vi "Find Average Center_10152025.vi"(5 "Position":i32, 7 "Tray Number":i32, 8 "Assembly Type":string, 9 "XYZTheta":dbl[](array[numeric]), 11 "Gantry In":refnum<k24>) -> (1 "XYZTheta":dbl[](array[numeric]) format="%.6g", 3 "Gantry Out":refnum<k24>)   [LabVIEW 2021, in "Component Tray.lvclass"]
uses:
  Component Tray.lvclass
  Find Component.ctl
  Controller/Camera/Machine Vision.ctl
  C:/Program Files (x86)/Aerotech/A3200/LabVIEW/2010/Bin/Aerotech.A3200.dll
  Program Files (x86)/Aerotech/A3200/LabVIEW/2010/Bin/Aerotech.A3200.dll
  Controller/Camera/Image processing.ctl
  Controller/Camera/Camera settings.ctl
  <vilib>/vision/Pattern Matching.llb/IMAQ GM Match Report.ctl
  Controller/Camera/Edmund Optics/Edmund Optics.lvclass
  C:/Users/HEP/Documents/GitHub/Gantry/UCSB-Gantry-HEP-main/Classes/Controller/Camera/Camera.lvclass
  <vilib>/picture/picture.llb/imagedata.ctl
  Controller/Camera/Camera.lvclass
  Controller/Motion/A3200/A3200.lvclass
  Controller/Motion/Motion.lvclass
panel:
  out "pattern matching":T1 {"Correlation Score" format="%.2f"; "Target Template Curve Score" format="%.2f"; "Template Target Curve Score" format="%.2f"; "Bounding Box"."y" format="%.2f"; "Bounding Box"."x" format="%.2f"; "Position"."y" format="%.2f"; "Position"."x" format="%.2f"; "Score" format="%.2f"; "Scale" format="%.2f"; "Angle" format="%.2f"; "Occlusion %" format="%.2f"}
  out "Maximal Value":sgl
  out "Standard Variation":sgl
  out "Match found?":bool
  out "Radius (Real-World)":dbl
  in  "Enter Manual Mode":bool
  out "Manual Mode On":bool
  in  "Auto Submit":bool
  out "Instructions":string="Use the joystick to match the pattern recognition until a red circle appears.\nUse Z controls to focus if needed."
  out "Tray and Position":string
  out "Sensor ID":picture[](array[picture])
  out "Sensor ID":string
  in  "Machine Vision":T2
  out "predicted fiducials":dbl[][](array[numeric])
  out "Current Z High Speed":dbl
  out "Current XY High Speed":dbl
  out "current Z low speed":dbl
  out "current XY speed":dbl
  in  "Z high":dbl=12.5
  in  "XY high":dbl=50.0
  in  "Z low":dbl=0.05
  in  "XY low":dbl=0.1
  in  "Predict fiducials":bool
  out "Low Speed":bool
  out "X":bool
  out "Y":bool
  out "Z":bool
  out "High Speed":bool
  in  "Go to CH191/FD5":bool
  in  "Go to CH197/FD4":bool
  out "Program Stopped":bool
  out "XY Graph":cluster{"X":dbl, "Y":dbl}[](graph)
  out "Sensor ID Location":dbl[](array[numeric])
  in  "Go to Sensor ID":bool
  out "CH1 XYZ":dbl[](array[numeric])
  out "CH1 correct?":bool
  in  "Go to CH1":bool
  in  "Focus step size":dbl format="%#_13g"
  in  "number of focus steps":i32
  out "Average Strength":dbl
  in  "Focus":bool
  out "All fiducials recorded":bool
  in  "Override presets":bool
  in  "Camera settings":T3={"Gamma"=1.6, "Gain"=0, "Sharpness"=0, "Contrast"=0.0, "Exposure"=0.0078125} {"Exposure" min=0.000244140625 max=0.5 scale=0.0002..0.5; "Contrast" min=0.0 max=1.0 scale=0.001..1.0; "Sharpness" min=0 max=2 step=1 scale=0.0..2.0; "Gain" min=0 max=100 step=1 scale=0.1..100.0; "Gamma" min=0.01 max=10.0 scale=0.01..10.0}
  in  "Image processing":T4={"Brightness"=128.0, "Contrast"=45.0, "Gamma"=1.0471123} {"Brightness" scale=0.0..400.0; "Contrast" scale=0.0..90.0; "Gamma" scale=0.005..5.0}
  out "Gantry":dbl[](array[numeric]) format="%.6g"
  out "Sum":dbl[](array[numeric]) format="%.6g"
  out "CH197/FD4 XYZ":dbl[](array[numeric]) format="%.6g"
  out "CH8/FD2 XYZ":dbl[](array[numeric]) format="%.6g"
  out "CH191/FD5 XYZ":dbl[](array[numeric]) format="%.6g"
  out "CH1/FD1 XYZ":dbl[](array[numeric]) format="%.6g"
  in  "Record CH8/FD2":bool
  in  "Record CH197/FD4":bool
  in  "Record CH191/FD5":bool
  in  "Record CH1/FD1":bool
  in  "Go to CH8/FD2":bool
  in  "Go to CH1/FD1":bool
  in  "Joystick":bool
  out "Camera":dbl[](array[numeric]) format="%.6g"
  in  "Go to Center":bool
  in  "Component":T5
  in  "Stop Program":bool
  out "Image":T6(plugin-control)
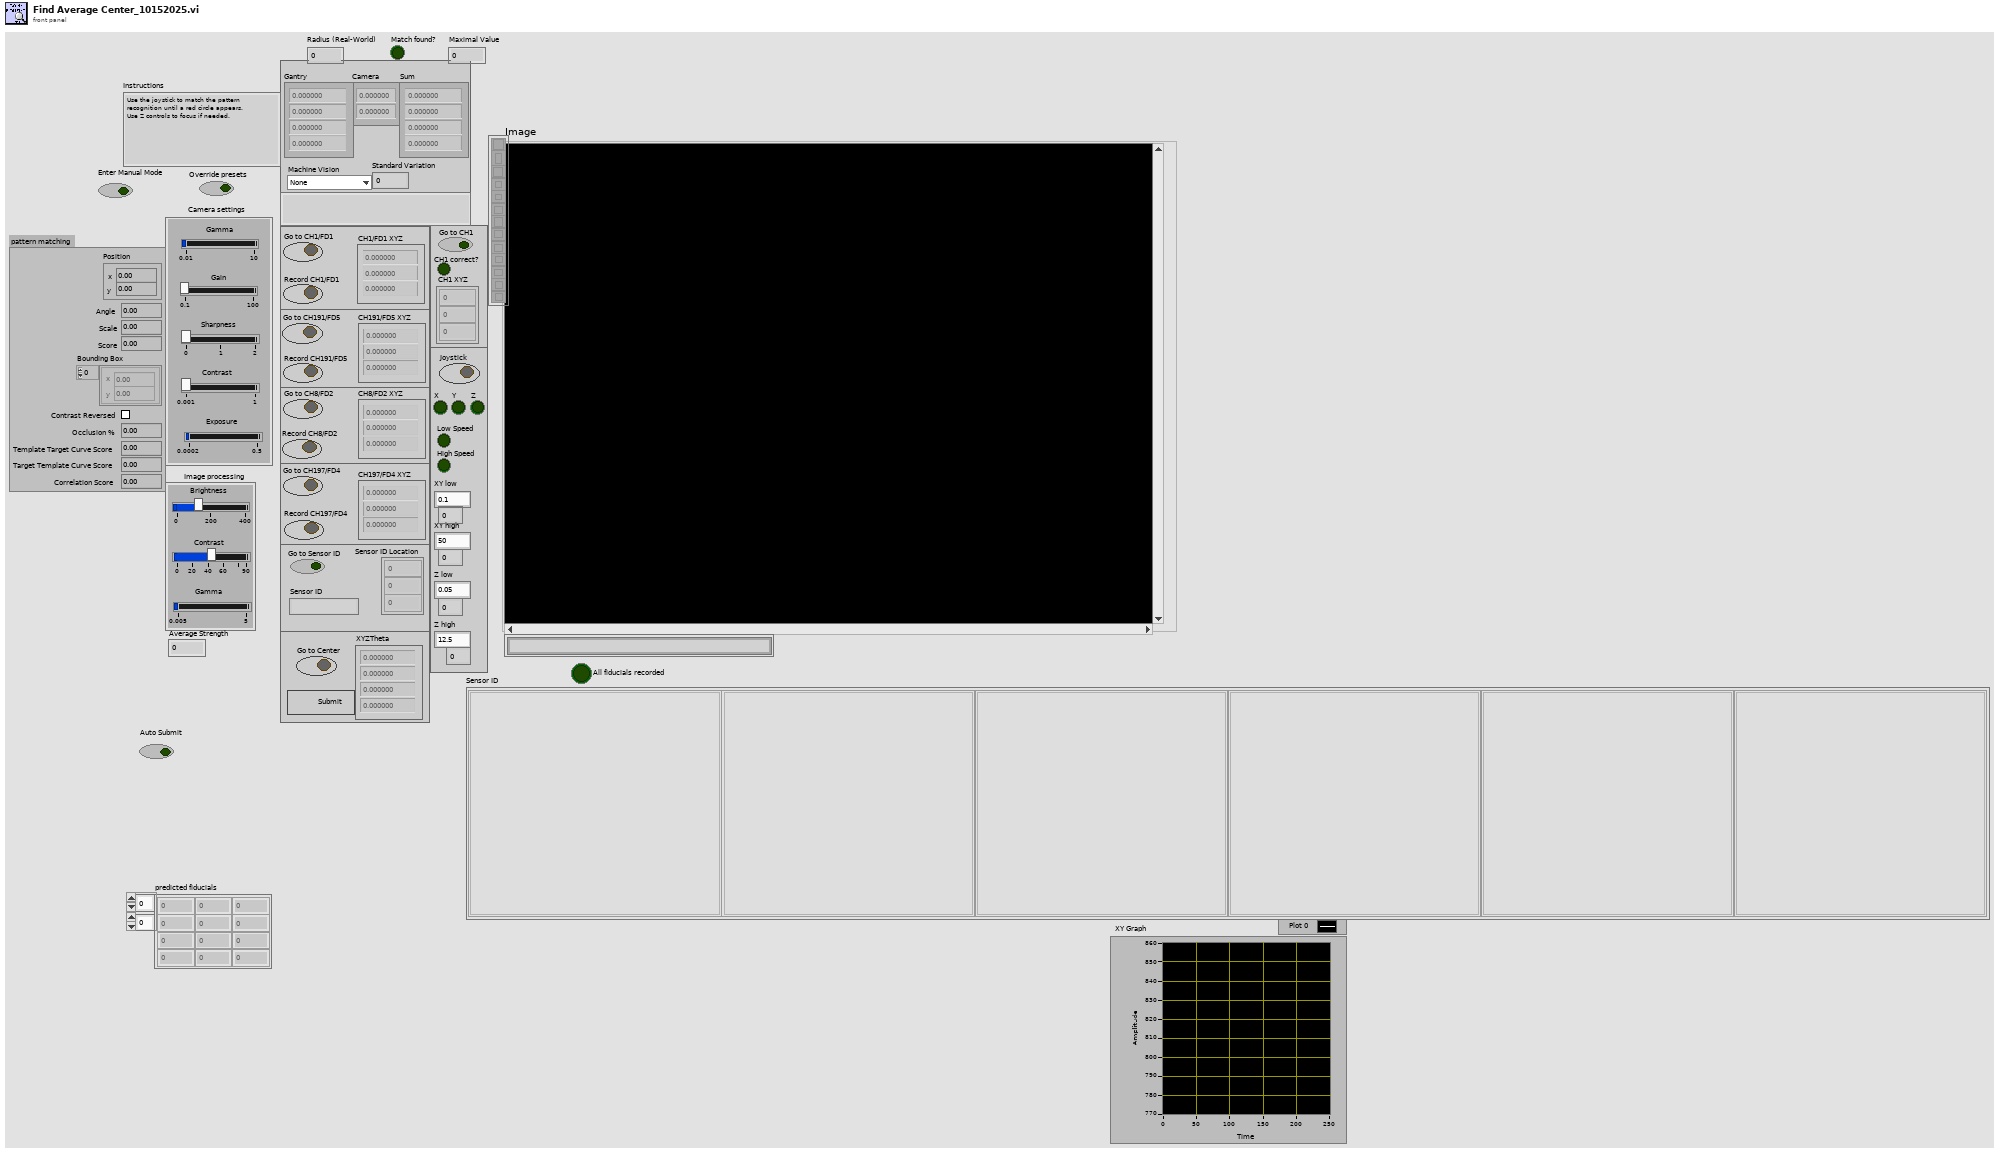
[diagram p1: front panel]
types:
  T1 = typedef "IMAQ GM Match Report.ctl" = cluster{"Position":cluster{"x":sgl, "y":sgl}, "Angle":sgl, "Scale":sgl, "Score":sgl, "Bounding Box":cluster{"x":sgl, "y":sgl}[], "Contrast Reversed":bool, "Occlusion %":sgl, "Template Target Curve Score":sgl, "Target Template Curve Score":sgl, "Correlation Score":sgl}
  T2 = typedef "Camera.lvclass/Machine Vision.ctl" = enum16{"None", "Tray Fiducials", "Sensor Fiducial", "V3 Sensor Circle", "Partial Hexaboard", "Hexaboard Circle", "sensor CH1 check", "sensor edge pos1", "sensor edge pos2", "HB edge pos1", "HB edge pos2", "HB Fiducial", "HB CH1 check "}
  T3 = typedef "Camera.lvclass/Camera settings.ctl" = cluster{"Gamma":dbl, "Gain":i64, "Sharpness":i64, "Contrast":dbl, "Exposure":dbl}
  T4 = typedef "Camera.lvclass/Image processing.ctl" = cluster{"Brightness":sgl, "Contrast":sgl, "Gamma":sgl}
  T5 = typedef "Component Tray.lvclass/Find Component.ctl" = cluster{"New Fiducials":dbl[], "Past Fiducials":dbl[][], "XYZTheta":dbl[], "Fiducials Path":path, "Position":i32, "CH1 Location":dbl[], "Sensor ID Location":dbl[], "raw rotation":dbl, "initial rotation":dbl[], "CH2":dbl[], "initial edge XYZ":dbl[], "max std variation":dbl, "max strength":dbl, "Pattern Matching":T2, "Fiducial Circle":T2, "Initial Edge":T2, "Pos multiplier":dbl, "time to wait":u32, "fiducial to edge":dbl, "Protomodule?":bool, "Assembly Type":string}
  T6 = typedef "IMAQ Image.ctl" = refnum<image>
  T7 = enum8{"Enabled", "Disabled", "Disabled and Grayed Out"}
  T8 = cluster{"left":i16, "top":i16, "right":i16, "bottom":i16}
  T9 = typedef "imagedata.ctl" = cluster{"image type":i32, "image depth":i32, "image":u8[], "mask":u8[], "colors":u32[], "Rectangle":cluster{"left":i16, "top":i16, "right":i16, "bottom":i16}}
  T10 = typedef "File Paths.ctl" = cluster{"Glue Pattern Folder":path, "Carrier Tray Folder":path, "Pick Up Tool Fixture Folder":path, "Components Folder":path, "Bellows Tool Offset.txt":path, "Pick Up Tool Offset.txt":path, "Dispense Tip Offset.txt":path, "Log Files":path, "Gantry Assembly Map.txt":path, "Syringe and offset map.txt":path, "Controllers Folder":path, "Local dbase config":path}
  T11 = cluster{"left":dbl, "top":dbl, "right":dbl, "bottom":dbl}
  T12 = cluster{"Average Strength":dbl, "Radius (Real-World)":dbl, "Match found?":bool, "initial angle":sgl, "Global Report":cluster{"Mean Value":sgl, "Standard Variation":sgl, "Minimal Value":sgl, "Maximal Value":sgl, "Area (calibrated)":sgl, "Area (pixels)":u32, "%":sgl, "Calibration Valid":bool}}
  T13 = cluster{"Mean Value":sgl, "Standard Variation":sgl, "Minimal Value":sgl, "Maximal Value":sgl, "Area (calibrated)":sgl, "Area (pixels)":u32, "%":sgl, "Calibration Valid":bool}
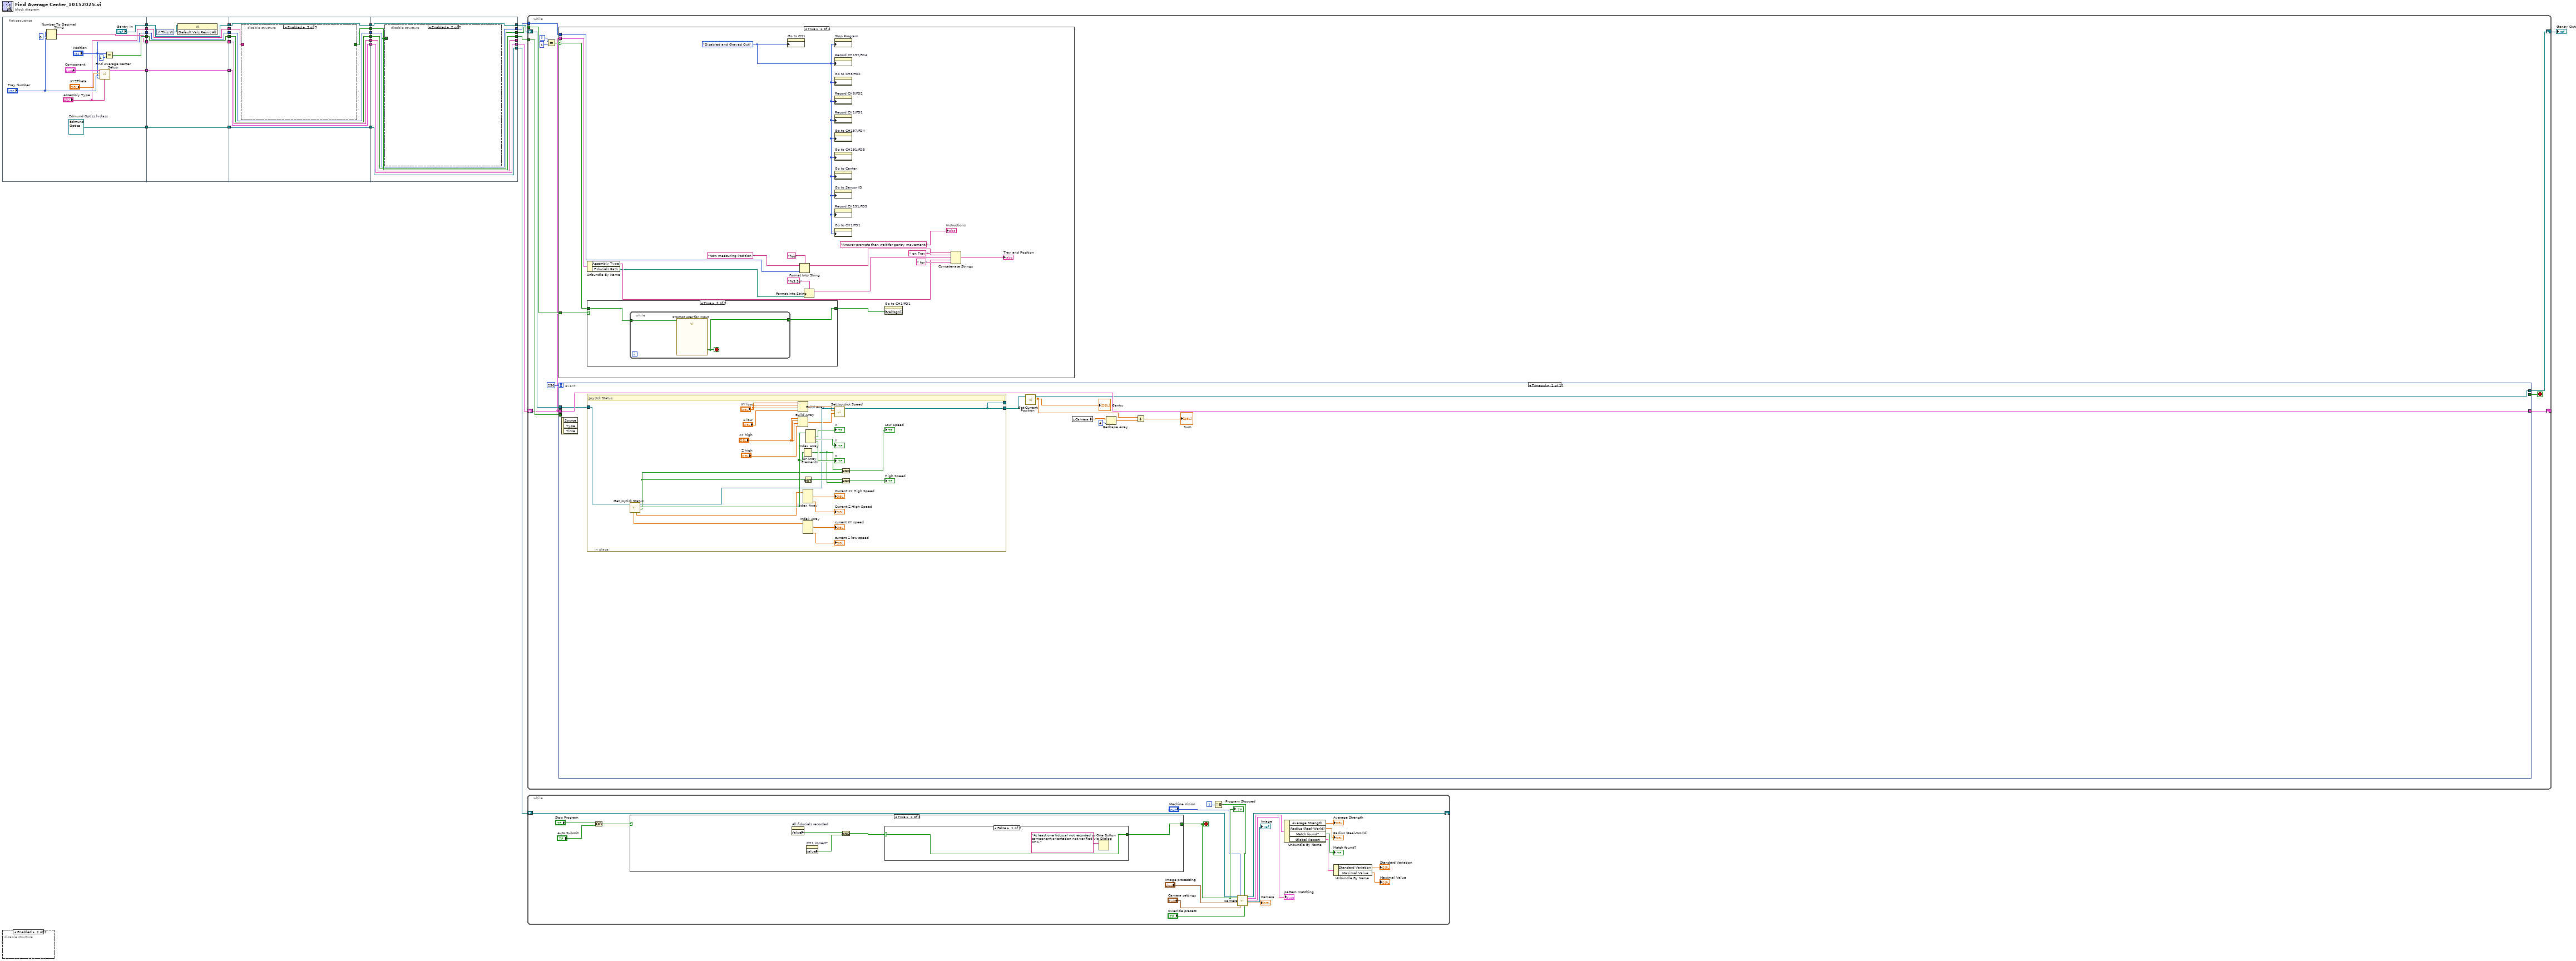
[diagram p0: block diagram]
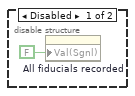
[diagram p2: hidden frame]
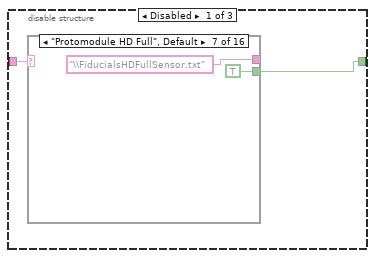
[diagram p3: hidden frame]
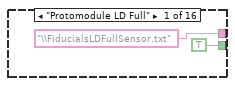
[diagram p4: hidden frame]
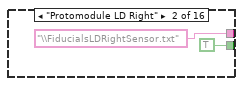
[diagram p5: hidden frame]
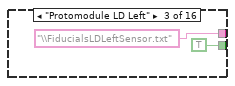
[diagram p6: hidden frame]
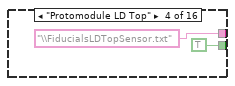
[diagram p7: hidden frame]
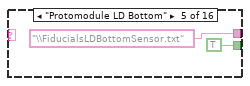
[diagram p8: hidden frame]
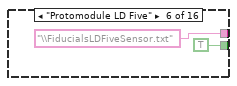
[diagram p9: hidden frame]
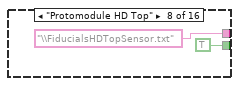
[diagram p10: hidden frame]
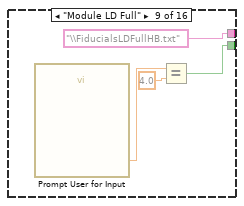
[diagram p11: hidden frame]
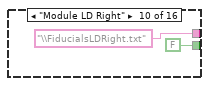
[diagram p12: hidden frame]
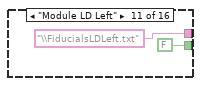
[diagram p13: hidden frame]
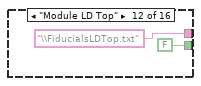
[diagram p14: hidden frame]
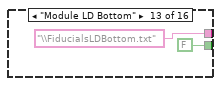
[diagram p15: hidden frame]
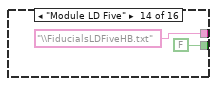
[diagram p16: hidden frame]
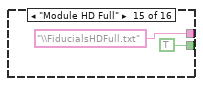
[diagram p17: hidden frame]
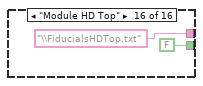
[diagram p18: hidden frame]
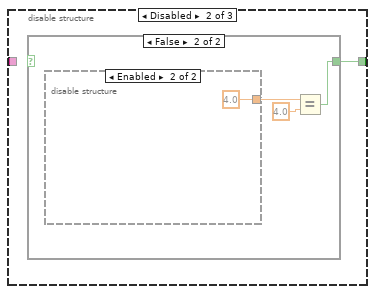
[diagram p19: hidden frame]
diagram:
  n1 = flat-sequence {
    tunnel: [w33] -> w23
    tunnel: [w37] -> w19
    tunnel: ["Gantry In"] -> w15
    tunnel: [w36] -> w12
    tunnel: ["Position"] -> w8
    tunnel: [w35] -> w5
    tunnel: ["Assembly Type"] -> w2
    tunnel: [w47] -> w24
    tunnel: w23 -> [w47]
    tunnel: [w46] -> w20
    tunnel: w19 -> [w46]
    tunnel: [w45] -> w16
    tunnel: w15 -> [w45]
    tunnel: [w44] -> w13
    tunnel: w12 -> [w44]
    tunnel: [w43] -> w9
    tunnel: w8 -> [w43]
    tunnel: w5 -> [w42]
    tunnel: [w42] -> w3
    tunnel: w2 -> [w41]
    tunnel: [w41] -> w1
    tunnel: [w56] -> w27
    tunnel: [w55] -> w25
    tunnel: w24 -> [w55]
    tunnel: [w54] -> w21
    tunnel: w20 -> [w54]
    tunnel: [w53] -> w17
    tunnel: w16 -> [w53]
    tunnel: w13 -> [w52]
    tunnel: [w52] -> w11
    tunnel: w9 -> [w51]
    tunnel: [w51] -> w7
    tunnel: [w50] -> w4
    tunnel: w3 -> [w50]
    tunnel: w1 -> [w49]
    tunnel: w27 -> [w106]
    tunnel: [w106] -> w26
    tunnel: [w105] -> w22
    tunnel: w25 -> [w105]
    tunnel: w21 -> [w104]
    tunnel: [w104] -> w18
    tunnel: [w103] -> w14
    tunnel: w17 -> [w103]
    tunnel: w11 -> [w102]
    tunnel: [w102] -> w10
    tunnel: [w101] -> w6
    tunnel: w7 -> [w101]
    tunnel: w4 -> [w100]
    tunnel: [w100] -> _
    frame #0 {
      w37 = refnum<class "Edmund Optics.lvclass"> refnum  # Edmund Optics.lvclass
      n2 = Number To Decimal String(number="Tray Number", width (-)=i16 0) -> (decimal integer string=w35:string)
      n3 = call "Find Average Center Setup.vi"("Assembly Type"="Assembly Type", "Position"="Position", "Tray Number"="Tray Number", "XYZTheta"="XYZTheta", "Component"="Component") -> ("output cluster"=w33:T5)  [unwired: 6 in]
      n4 = Equal?(x="Position", y=1) -> (x = y?=w36:bool)
    }
    frame #1 {
      n5 = control-ref of="This VI"() -> (w48:refnum<vi>)
      n6 = invoke class="VI" method="Default Vals.Reinit All"(reference=w48) -> ()  [unwired: 2 in, 3 out]
    }
    frame #2 {
      n7 = disable-structure shown="Enabled" {
        disable-tunnel: [w58 w93 _] -> w56
        disable-tunnel: w49 -> [w57 _ _]
        frame Disabled {
          n8 = case shown="\"Protomodule HD Full\", Default" w57 {
            tunnel: ["\\FiducialsLDFullSensor.txt" ("string") "\\FiducialsLDRightSensor.txt" ("string") "\\FiducialsLDLeftSensor.txt" ("string") "\\FiducialsLDTopSensor.txt" ("string") "\\FiducialsLDBottomSensor.txt" ("string") "\\FiducialsLDFiveSensor.txt" ("string") "\\FiducialsHDFullSensor.txt" ("string") "\\FiducialsHDTopSensor.txt" ("string") "\\FiducialsLDFullHB.txt" ("string") "\\FiducialsLDRight.txt" ("string") "\\FiducialsLDLeft.txt" ("string") "\\FiducialsLDTop.txt" ("string") "\\FiducialsLDBottom.txt" ("string") "\\FiducialsLDFiveHB.txt" ("string") "\\FiducialsHDFull.txt" ("string") "\\FiducialsHDTop.txt" ("string")] -> _
            tunnel: [TRUE TRUE TRUE TRUE TRUE TRUE TRUE TRUE w75 FALSE FALSE FALSE FALSE FALSE TRUE FALSE] -> w58
            frame "Protomodule LD Full" {
            }
            frame "Protomodule LD Right" {
            }
            frame "Protomodule LD Left" {
            }
            frame "Protomodule LD Top" {
            }
            frame "Protomodule LD Bottom" {
            }
            frame "Protomodule LD Five" {
            }
            frame "Protomodule HD Full", Default {
            }
            frame "Protomodule HD Top" {
            }
            frame "Module LD Full" {
              n9 = call "Prompt User for Input"() -> ("NumFD"=w77:dbl)  [unwired: 17 in, 2 out]
              n10 = Equal?(x=w77, y=4.0) -> (x = y?=w75:bool)
            }
            frame "Module LD Right" {
            }
            frame "Module LD Left" {
            }
            frame "Module LD Top" {
            }
            frame "Module LD Bottom" {
            }
            frame "Module LD Five" {
            }
            frame "Module HD Full" {
            }
            frame "Module HD Top" {
            }
          }
        }
        frame Disabled {
          n11 = case shown="False" {
            selector: _ -> [w94 _]
            tunnel: [w94 w95] -> w93
            frame True {
            }
            frame False {
              n12 = disable-structure shown="Enabled" {
                disable-tunnel: [w98 4.0 ("NumFD")] -> w97
                frame Disabled {
                  n13 = call "Prompt User for Input2"() -> ("NumFD"=w98:dbl)  [unwired: 17 in, 2 out]
                }
                frame Enabled {
                }
              }
              n14 = Equal?(x=w97, y=4.0) -> (x = y?=w95:bool)
            }
          }
        }
        frame Enabled {
        }
      }
    }
    frame #3 {
      n15 = disable-structure shown="Enabled" {
        disable-tunnel: w106 -> [w107 _]
        frame Disabled {
          n16 = Select(t=T7."Enabled" ("Disabled"), s=w107, f=T7."Disabled and Grayed Out" ("Disabled")) -> (s? t:f=w108:T7)
          n17 = property on="Predict fiducials" class="Bool (strict)"("DisabledEnum"=w108) -> ()  [unwired: 2 in, 2 out]
          n18 = property on="Record CH197/FD4" class="Bool (strict)"("DisabledEnum"=w108) -> ()  [unwired: 2 in, 2 out]
          n19 = property on="Go to CH197/FD4" class="Bool (strict)"("DisabledEnum"=w108) -> ()  [unwired: 2 in, 2 out]
          n20 = property on="CH197/FD4 XYZ" class="Arr (strict)"("DisabledEnum"=w108) -> ()  [unwired: 2 in, 2 out]
          n21 = property on="Record CH191/FD5" class="Bool (strict)"("DisabledEnum"=w108) -> ()  [unwired: 2 in, 2 out]
          n22 = property on="CH191/FD5 XYZ" class="Arr (strict)"("DisabledEnum"=w108) -> ()  [unwired: 2 in, 2 out]
          n23 = property on="Go to CH191/FD5" class="Bool (strict)"("DisabledEnum"=w108) -> ()  [unwired: 2 in, 2 out]
        }
        frame Enabled {
        }
      }
    }
  }
  n24 = disable-structure shown="Enabled" {
    frame Disabled {
      n25 = property on="All fiducials recorded" class="Bool (strict)"("Val(Sgnl)"=FALSE) -> ()  [unwired: 2 in, 2 out]
    }
    frame Enabled {
    }
  }
  n26 = while {
    shift-right: [w122] -> _
    shift-left: w22 -> [w112]
    shift-right: [w119] -> w28
    shift-left: w14 -> [w120]
    tunnel: w26 -> [w118]
    tunnel: w10 -> [w114]
    tunnel: w6 -> [w113]
    i -> [w117]
    stop <- w123 stop-if-true
    n27 = Equal?(x=w117, y=1) -> (x = y?=w115:bool)
    n28 = case shown="True" w115 {
      selector: w115 -> [_ w138]
      tunnel: w114 -> [_ w137]
      tunnel: w113 -> [_ w136]
      tunnel: w112 -> [_ w128]
      frame False {
      }
      frame True {
        w133 = T7."Disabled and Grayed Out" ("Disabled")
        n29 = Unbundle By Name(w128) -> ("Assembly Type"=w127:string, "Fiducials Path"=w126:path)
        n30 = case shown="True" w137 {
          tunnel: [w141 w143] -> w140
          tunnel: w138 -> [w141 w142]
          frame False {
          }
          frame True {
            n31 = while {
              tunnel: [w145] -> w143
              tunnel: w142 -> [w144]
              stop <- w145 stop-if-true
              n32 = call "Prompt User for Input"("Enable"=w144) -> ("Sensors inspected?"=w145:bool)  [unwired: 16 in, 2 out]
            }
          }
        }
        n33 = property on="Go to CH1" class="Bool (strict)"("DisabledEnum"=w133) -> ()  [unwired: 2 in, 2 out]
        n34 = Format Into String(format string="%d", initial string="Now measuring Position ", w136) -> (resulting string=w132:string)  [unwired: 1 in, 1 out]
        n35 = Format Into String(format string="%3.3s", w126) -> (resulting string=w124:string)  [unwired: 2 in, 1 out]
        n36 = property on="Stop Program" class="Bool"("DisabledEnum"=w133) -> ()  [unwired: 2 in, 2 out]
        n37 = property on="Record CH197/FD4" class="Bool (strict)"("DisabledEnum"=w133) -> ()  [unwired: 2 in, 2 out]
        n38 = property on="Go to CH8/FD2" class="Bool (strict)"("DisabledEnum"=w133) -> ()  [unwired: 2 in, 2 out]
        n39 = property on="Record CH8/FD2" class="Bool (strict)"("DisabledEnum"=w133) -> ()  [unwired: 2 in, 2 out]
        n40 = property on="Record CH1/FD1" class="Bool (strict)"("DisabledEnum"=w133) -> ()  [unwired: 2 in, 2 out]
        n41 = property on="Go to CH197/FD4" class="Bool (strict)"("DisabledEnum"=w133) -> ()  [unwired: 2 in, 2 out]
        n42 = property on="Go to CH191/FD5" class="Bool (strict)"("DisabledEnum"=w133) -> ()  [unwired: 2 in, 2 out]
        n43 = property on="Go to Center" class="Bool"("DisabledEnum"=w133) -> ()  [unwired: 2 in, 2 out]
        n44 = property on="Go to Sensor ID" class="Bool (strict)"("DisabledEnum"=w133) -> ()  [unwired: 2 in, 2 out]
        n45 = property on="Record CH191/FD5" class="Bool (strict)"("DisabledEnum"=w133) -> ()  [unwired: 2 in, 2 out]
        n46 = property on="Go to CH1/FD1" class="Bool (strict)"("DisabledEnum"=w133) -> ()  [unwired: 2 in, 2 out]
        n47 = property on="Go to CH1/FD1" class="Bool (strict)"("Val(Sgnl)"=w140) -> ()  [unwired: 2 in, 2 out]
        n48 = Concatenate Strings(w132, " on Tray " ("string"), w124, " for " ("string"), w127) -> (→"Tray and Position":string)
        "Instructions" <- "Answer prompts then wait for gantry movement." ("Instructions")
      }
    }
    n49 = event shown="[0] Timeout" {
      selector: _ -> [_ _ _ _ _ _ _ _ _ _ _]
      dyn-events: _ -> [_ _ _ _ _ _ _ _ _ _ _]
      timeout: 250 -> [_ _ _ _ _ _ _ _ _ _ _]
      tunnel: [_ w182 _ _ _ _ _ _ _ _ _] -> w123
      tunnel: w112 -> [w153 w184 w210 w354 w522 w571 w617 w625 w650 w675 w688]
      tunnel: [w153 w184 w211 w359 w521 w571 w617 w625 w650 w675 w688] -> w122
      tunnel: w120 -> [w147 w185 w220 w383 w528 w573 w616 w621 w646 w676 w687]
      tunnel: [w149 w183 w224 w381 w528 w572 w614 w619 w644 w676 w686] -> w119
      tunnel: w118 -> [_ _ _ w374 _ _ _ _ _ w677 _]
      event Timeout {
        n50 = event-data() -> ()  [unwired: 1 in, 3 out]
        n51 = in-place {
          in-place-border: w147 -> [w178]
          in-place-border: [w167] -> _
          in-place-border: [w167] -> w146
          # "Joystck Status"
          n52 = call "Get Joytick Status.vi"("Gantry In"=w178) -> ("JoystickLowSpeedActive"=w172:bool, "Joystick Status"=w174:bool[], "Gantry Out"=w168:refnum<k24>, "High Speeds"=w156:dbl[], "Low Speeds"=w155:dbl[])  [unwired: 5 in, 1 out]
          n53 = Build Array("XY low", "XY low", "XY low", "Z low") -> (w162:dbl[])
          n54 = Build Array("XY high", "XY high", "XY high", "Z high") -> (w161:dbl[])
          n55 = Or Array Elements(Boolean array=w174) -> (logical OR=w170:bool)
          n56 = Not(x=w172) -> (.not. x?=w171:bool)
          n57 = Index Array(array=w156) -> (element #1=→"Current XY High Speed":dbl, element #3=→"Current Z High Speed":dbl)  [unwired: 3 in, 1 out]
          n58 = Index Array(array=w155) -> (element #1=→"current XY speed":dbl, element #3=→"current Z low speed":dbl)  [unwired: 3 in, 1 out]
          n59 = Index Array(array=w174) -> (element #1=→"X":bool, element #2=→"Y":bool, element #3=→"Z":bool)  [unwired: 3 in]
          n60 = call "Set Joystick Speed.vi"("High Speed Inputs"=w161, "Low Speed Inputs"=w162, "Gantry"=w168) -> ("Controller Out"=w167:refnum<k24>)  [unwired: 7 in, 1 out]
          n61 = And(x=w170, y=w172) -> (x .and. y?=→"Low Speed":bool)
          n62 = And(x=w171, y=w170) -> (x .and. y?=→"High Speed":bool)
        }
        n63 = call "Get Current Position.vi"("Gantry In"=w146) -> ("XYZTheta Out"=w148:dbl[], "Gantry Out"=w149:refnum<k24>)  [unwired: 8 in, 1 out]
        "Gantry" <- w148
        n64 = local read "Camera"() -> (w152:dbl[])
        n65 = Reshape Array(w152, 4 ("dimension size")) -> (w150:dbl[])
        n66 = Add(x=w148, y=w150) -> (x+y=→"Sum":dbl[])
      }
      event "Stop Program", "Auto Submit": Value Change {
        n67 = event-data() -> ()  [unwired: 1 in, 6 out]
        n68 = property on="All fiducials recorded" class="Bool (strict)"() -> ("Value"=w180:bool)  [unwired: 2 in, 2 out]
        n69 = property on="CH1 correct?" class="Bool (strict)"() -> ("Value"=w181:bool)  [unwired: 2 in, 2 out]
        n70 = And(x=w180, y=w181) -> (x .and. y?=w179:bool)
        n71 = case shown="True" w179 {
          selector: w179 -> [w186 w200]
          tunnel: w185 -> [w187 w202]
          tunnel: w184 -> [_ w203]
          tunnel: [w187 w201] -> w183
          tunnel: [w186 w200] -> w182
          frame False {
          }
          frame True {
            n72 = Unbundle By Name(w203) -> ("Fiducials Path"=w199:path, "New Fiducials"=w198:dbl[], "Position"=w188:i32)
            n73 = call "Base File Path.vi"() -> ("Paths Out"=w193:T10)  [unwired: 11 in]
            n74 = Unbundle By Name(w193) -> ("Components Folder"=w191:path)
            n75 = call "Replace Row In File.vi"("Index"=w188, "Insert Array"=w198, "Path"=w199) -> ()  [unwired: 8 in, 1 out]
            n76 = control-ref of="Joystick"() -> (w196:refnum<vi>)
            n77 = String To Path(string="temp") -> (path=w192:path)
            n78 = property class="Bool (strict)"(reference=w196) -> (reference out=w195:refnum<vi>, "Value"=w197:bool)  [unwired: 1 in, 1 out]
            n79 = Build Path(base path=w191, name or relative path=w192) -> (appended path=w194:path)
            n80 = case shown="True" w197 {
              selector: w197 -> [_ w209]
              tunnel: w202 -> [w204 w208]
              tunnel: [w204 w207] -> w201
              tunnel: w195 -> [_ w205]
              frame False {
              }
              frame True {
                n81 = Not(x=w209) -> (.not. x?=w206:bool)
                n82 = call "Joystick.vi"("Joystick"=w206, "Gantry In"=w208) -> ("Gantry Out"=w207:refnum<k24>)  [unwired: 8 in, 1 out]
                n83 = property class="Bool (strict)"(reference=w205, "Value"=w206) -> ()  [unwired: 1 in, 2 out]
              }
            }
            n84 = Delete(path (use dialog)=w194, entire hierarchy (F)=TRUE) -> ()  [unwired: 3 in, 3 out]
          }
        }
      }
      event "Go to CH1/FD1", "Go to CH8/FD2", "Go to CH197/FD4", "Go to CH191/FD5": Value Change {
        n85 = event-data() -> ()  [unwired: 1 in, 6 out]
        n86 = flat-sequence {
          tunnel: w220 -> [w230]
          tunnel: [w230] -> w219
          tunnel: [w225] -> w214
          tunnel: [w237] -> w218
          tunnel: w219 -> [w244]
          tunnel: [w234] -> w216
          tunnel: [w239] -> w215
          tunnel: [w238] -> w217
          tunnel: w214 -> [w235]
          tunnel: [w234] -> w213
          tunnel: w210 -> [w233]
          tunnel: [w249] -> w223
          tunnel: w218 -> [w251]
          tunnel: w217 -> [w250]
          tunnel: w216 -> [w248]
          tunnel: w215 -> [w246]
          tunnel: [w245] -> w212
          tunnel: w223 -> [w269]
          tunnel: [w268] -> w222
          tunnel: w210 -> [w270]
          tunnel: w212 -> [w267]
          tunnel: w210 -> [w266]
          tunnel: [w265] -> w211
          tunnel: [w341] -> w224
          tunnel: w222 -> [w341]
          tunnel: w213 -> [w340]
          tunnel: w221 -> [w339]
          frame #0 {
            n87 = Build Array "Build Array"("Go to CH1/FD1", "Go to CH191/FD5", "Go to CH8/FD2", "Go to CH197/FD4") -> (w225:bool[])
          }
          frame #1 {
            w241 = T7."Disabled and Grayed Out" ("Disabled")
            w243 = FALSE ("Go to Top Right Fiducial")
            n88 = Unbundle By Name(w233) -> ("Past Fiducials"=w232:dbl[][], "Pattern Matching"=w231:T2)
            n89 = Search 1D Array(1D array=w235, element=TRUE) -> (index of element=w234:i32)  [unwired: 1 in]
            n90 = property on="Go to CH1/FD1" class="Bool (strict)"("Value"=w243) -> ()  [unwired: 2 in, 2 out]
            n91 = property on="Go to CH191/FD5" class="Bool (strict)"("Value"=w243) -> ()  [unwired: 2 in, 2 out]
            n92 = property on="Go to CH8/FD2" class="Bool (strict)"("Value"=w243) -> ()  [unwired: 2 in, 2 out]
            n93 = property on="Go to CH197/FD4" class="Bool (strict)"("Value"=w243) -> ()  [unwired: 2 in, 2 out]
            n94 = local write "Machine Vision"(w231) -> ()
            n95 = Index Array(array=w232, index (row)=w234) -> (element=w237:dbl[])  [unwired: 1 in]
            n96 = property on="Instructions" class="Str"("Val(Sgnl)"="Wait for movement to stop." ("Value (Signaling)")) -> ()  [unwired: 2 in, 2 out]
            n97 = property on="Go to CH1/FD1" class="Bool (strict)"("DisabledEnum"=w241) -> ()  [unwired: 2 in, 2 out]
            n98 = property on="Record CH1/FD1" class="Bool (strict)"("DisabledEnum"=w241) -> ()  [unwired: 2 in, 2 out]
            n99 = property on="Go to CH1" class="Bool (strict)"("DisabledEnum"=w241) -> ()  [unwired: 2 in, 2 out]
            n100 = property on="Go to CH191/FD5" class="Bool (strict)"("DisabledEnum"=w241) -> ()  [unwired: 2 in, 2 out]
            n101 = property on="Record CH191/FD5" class="Bool (strict)"("DisabledEnum"=w241) -> ()  [unwired: 2 in, 2 out]
            n102 = property on="Go to CH197/FD4" class="Bool (strict)"("DisabledEnum"=w241) -> ()  [unwired: 2 in, 2 out]
            n103 = property on="Record CH197/FD4" class="Bool (strict)"("DisabledEnum"=w241) -> ()  [unwired: 2 in, 2 out]
            n104 = property on="Go to CH8/FD2" class="Bool (strict)"("DisabledEnum"=w241) -> ()  [unwired: 2 in, 2 out]
            n105 = property on="Record CH8/FD2" class="Bool (strict)"("DisabledEnum"=w241) -> ()  [unwired: 2 in, 2 out]
            n106 = property on="Go to Center" class="Bool"("DisabledEnum"=w241) -> ()  [unwired: 2 in, 2 out]
            n107 = property on="Stop Program" class="Bool"("DisabledEnum"=w241) -> ()  [unwired: 2 in, 2 out]
            n108 = property on="Go to Sensor ID" class="Bool (strict)"("DisabledEnum"=w241) -> ()  [unwired: 2 in, 2 out]
            n109 = call "Joystick.vi"("Joystick"=FALSE, "Gantry In"=w244) -> ("error out"=w239:errorcluster, "Gantry Out"=w238:refnum<k24>)  [unwired: 8 in]
          }
          frame #2 {
            n110 = Equal To 0?(x=w248) -> (x = 0?=w247:bool)
            n111 = case shown="False" w247 {
              tunnel: w251 -> [w254 w264]
              tunnel: w250 -> [w259 w263]
              tunnel: [w258 w262] -> w249
              tunnel: w246 -> [w256 w260]
              tunnel: [w252 w261] -> w245
              frame False {
                w257 = FALSE ("Increment?")
                n112 = Array Subset(array=w254) -> (w253:dbl[])  [unwired: 2 in]
                n113 = call "XY Go.vi"("Increment?"=w257, "return immediately"=w257, "error in (no error)"=w256, "Speed"=300.0, "XY In"=w253, "Gantry In"=w259) -> ("error out"=w252:errorcluster, "Gantry Out"=w258:refnum<k24>)  [unwired: 3 in, 1 out]
              }
              frame True {
                n114 = call "ClearXYZTheta Go.vi"("error in (no error)"=w260, "XYZTheta In"=w264, "Gantry In"=w263) -> ("error out"=w261:errorcluster, "Gantry Out"=w262:refnum<k24>)  [unwired: 6 in, 1 out]
              }
            }
          }
          frame #3 {
            n115 = flat-sequence {
              tunnel: w270 -> [w272]
              tunnel: w269 -> [w277]
              tunnel: [w276] -> w268
              tunnel: w267 -> [w275]
              tunnel: w266 -> [w274]
              tunnel: [w273] -> w265
              frame #0 {
                n116 = Unbundle By Name(w272) -> ("time to wait"=w271:u32)
                n117 = Wait (ms)(milliseconds to wait=w271) -> ()  [unwired: 1 out]
              }
              frame #1 {
                n118 = local read "Match found?"() -> (w278:bool)
                n119 = case shown="True" w278 {
                  tunnel: w277 -> [w281 w296]
                  tunnel: [w281 w295] -> w276
                  tunnel: w275 -> [w279 w294]
                  tunnel: w274 -> [w280 w286]
                  tunnel: [w279 w288] -> _
                  tunnel: [w280 w287] -> w273
                  frame False {
                  }
                  frame True {
                    n120 = Unbundle By Name(w286) -> ("time to wait"=w282:u32, "Fiducial Circle"=w291:T2)
                    n121 = flat-sequence {
                      tunnel: w296 -> [w304]
                      tunnel: w294 -> [w300]
                      tunnel: [w303] -> w293
                      tunnel: w291 -> [w298]
                      tunnel: [w297] -> w290
                      tunnel: w293 -> [w307]
                      tunnel: w282 -> [w306]
                      tunnel: [w307] -> w292
                      tunnel: w290 -> [w305]
                      tunnel: [w305] -> w289
                      tunnel: w292 -> [w313]
                      tunnel: w289 -> [w311]
                      tunnel: w286 -> [w308]
                      tunnel: [w312] -> w285
                      tunnel: [w310] -> w284
                      tunnel: [w309] -> w283
                      tunnel: [w336] -> w287
                      tunnel: [w337] -> w288
                      tunnel: [w338] -> w295
                      tunnel: w285 -> [w338]
                      tunnel: w284 -> [w337]
                      tunnel: w283 -> [w336]
                      tunnel: w282 -> [w335]
                      frame #0 {
                        n122 = local write "Machine Vision"(w298) -> ()
                        n123 = local read "Camera"() -> (w302:dbl[])
                        n124 = call "XY Go.vi"("Increment?"=TRUE, "error in (no error)"=w300, "Speed"=1.0, "XY In"=w302, "Gantry In"=w304) -> ("error out"=w297:errorcluster, "Gantry Out"=w303:refnum<k24>)  [unwired: 4 in, 1 out]
                      }
                      frame #1 {
                        n125 = Wait (ms)(milliseconds to wait=w306) -> ()  [unwired: 1 out]
                      }
                      frame #2 {
                        n126 = in-place {
                          in-place-border: w313 -> [w323]
                          in-place-border: [w322] -> w312
                          in-place-border: w311 -> [w321]
                          in-place-border: [w320] -> w310
                          n127 = in-place-cluster #1(w308) -> ("max strength"=w314:dbl)
                          n128 = Subtract(x=w314, y=10.0) -> (x-y=w319:dbl)
                          n129 = local read "Average Strength"() -> (w315:dbl)
                          n130 = Less?(x=w315, y=w319) -> (x < y?=w317:bool)
                          n131 = case shown="False" w317 {
                            tunnel: w323 -> [w325 w334]
                            tunnel: [w325 w333] -> w322
                            tunnel: w321 -> [w324 w332]
                            tunnel: [w324 w331] -> w320
                            tunnel: [w326 w330] -> w316
                            tunnel: w315 -> [w328 _]
                            tunnel: w314 -> [w327 _]
                            frame False {
                              n132 = Greater?(x=w328, y=w327) -> (0:w329:bool)
                              n133 = Select(t=w328, s=w329, f=w327) -> (s? t:f=w326:dbl)
                            }
                            frame True {
                              n134 = call "Focus Strength.vi"("Gantry In"=w334, "error in"=w332) -> ("Gantry Out"=w333:refnum<k24>, "max value"=w330:dbl, "error out"=w331:errorcluster)  [unwired: 5 in]
                            }
                          }
                          n135 = in-place-cluster #1("max strength"=w316) -> (w309:T5)
                        }
                      }
                      frame #3 {
                        n136 = Wait (ms)(milliseconds to wait=w335) -> ()  [unwired: 1 out]
                      }
                    }
                  }
                }
              }
            }
          }
          frame #4 {
            n137 = case shown="False" w339 {
              tunnel: w340 -> [w342 _]
              frame False {
                n138 = case shown="0, Default" w342 {
                  frame 0, Default {
                    n139 = property on="Record CH1/FD1" class="Bool (strict)"("DisabledEnum"=T7."Enabled" ("Disabled")) -> ()  [unwired: 2 in, 2 out]
                    n140 = property on="Instructions" class="Str"("Val(Sgnl)"="Use the joystick to match the pattern recognition until a stable red circle appears. \nUse Z controls to focus or override camera presets if needed. \nClick Record CH1/FD1.") -> ()  [unwired: 2 in, 2 out]
                  }
                  frame 1 {
                    n141 = property on="Record CH191/FD5" class="Bool (strict)"("DisabledEnum"=T7."Enabled" ("Disabled")) -> ()  [unwired: 2 in, 2 out]
                    n142 = property on="Instructions" class="Str"("Val(Sgnl)"="Use the joystick to match the pattern recognition until a stable red circle appears. \nUse Z controls to focus or override camera presets if needed. \nClick Record CH191/FD5.") -> ()  [unwired: 2 in, 2 out]
                  }
                  frame 2 {
                    n143 = property on="Record CH8/FD2" class="Bool (strict)"("DisabledEnum"=T7."Enabled" ("Disabled")) -> ()  [unwired: 2 in, 2 out]
                    n144 = property on="Instructions" class="Str"("Val(Sgnl)"="Use the joystick to match the pattern recognition until a stable red circle appears. \nUse Z controls to focus or override camera presets if needed. \nClick Record CH8/FD2.") -> ()  [unwired: 2 in, 2 out]
                  }
                  frame 3 {
                    n145 = property on="Record CH197/FD4" class="Bool (strict)"("DisabledEnum"=T7."Enabled" ("Disabled")) -> ()  [unwired: 2 in, 2 out]
                    n146 = property on="Instructions" class="Str"("Val(Sgnl)"="Use the joystick to match the pattern recognition until a stable red circle appears. \nUse Z controls to focus or override camera presets if needed. \nClick Record CH197/FD4.") -> ()  [unwired: 2 in, 2 out]
                  }
                }
              }
              frame True {
                n147 = property on="Enter Manual Mode" class="Bool (strict)"("Val(Sgnl)"=TRUE ("Value (Signaling)")) -> ()  [unwired: 2 in, 2 out]
              }
            }
          }
        }
        n148 = property on="All fiducials recorded" class="Bool (strict)"() -> ("Value"=w221:bool)  [unwired: 2 in, 2 out]
      }
      event "Record CH1/FD1", "Record CH191/FD5", "Record CH197/FD4", "Record CH8/FD2": Value Change {
        n149 = event-data() -> ()  [unwired: 1 in, 1 out]
        n150 = flat-sequence {
          tunnel: [w397] -> w357
          tunnel: ["Record CH1/FD1"] -> w356
          tunnel: [w402] -> w376
          tunnel: w357 -> [w402]
          frame #0 {
            n151 = Build Array "Build Array"("Record CH1/FD1", "Record CH191/FD5", "Record CH8/FD2", "Record CH197/FD4") -> (w396:bool[])
            n152 = Search 1D Array(1D array=w396, element=TRUE) -> (index of element=w397:i32)  [unwired: 1 in]
          }
          frame #1 {
            w401 = FALSE ("Record CH1/FD1")
            n153 = property on="Record CH1/FD1" class="Bool (strict)"("Value"=w401) -> ()  [unwired: 2 in, 2 out]
            n154 = property on="Record CH191/FD5" class="Bool (strict)"("Value"=w401) -> ()  [unwired: 2 in, 2 out]
            n155 = property on="Record CH197/FD4" class="Bool (strict)"("Value"=w401) -> ()  [unwired: 2 in, 2 out]
            n156 = property on="Record CH8/FD2" class="Bool (strict)"("Value"=w401) -> ()  [unwired: 2 in, 2 out]
          }
        }
        n157 = call "Get Current Position.vi"("Gantry In"=w383) -> ("XYZTheta Out"=w382:dbl[], "Gantry Out"=w381:refnum<k24>)  [unwired: 8 in, 1 out]
        n158 = local read "Camera"() -> (w385:dbl[])
        n159 = Reshape Array(w385, 3 ("dimension size")) -> (w384:dbl[])
        n160 = Add(x=w382, y=w384) -> (x+y=w353:dbl[])
        n161 = control-ref of="CH191/FD5 XYZ"() -> (w379:refnum<vi>)
        n162 = control-ref of="CH197/FD4 XYZ"() -> (w377:refnum<vi>)
        n163 = control-ref of="CH1/FD1 XYZ"() -> (w380:refnum<vi>)
        n164 = control-ref of="CH8/FD2 XYZ"() -> (w378:refnum<vi>)
        n165 = case shown="True" w356 {
          tunnel: w354 -> [w390 w393]
          tunnel: [w390 w392] -> w355
          tunnel: w353 -> [_ w391]
          frame False {
          }
          frame True {
            n166 = call "Get Angle.vi"("array"=w391, "input cluster"=w393) -> ("output cluster"=w392:T5)  [unwired: 9 in]
          }
        }
        n167 = Build Array "Build Array"(w380, w379, w378, w377) -> (w389:refnum<vi>[])
        n168 = Index Array "Index Array"(array=w389, index=w376) -> (element=w388:refnum<vi>)
        n169 = Unbundle By Name(w355) -> ("New Fiducials"=w363:dbl[], "XYZTheta"=w373:dbl[], "Position"=w361:i32, "Assembly Type"=w352:string)  [unwired: 2 out]
        n170 = Multiply(x=w376, y=3) -> (x*y=w386:i32)
        n171 = case shown="False" w374 {
          selector: w374 -> [w403 w410]
          tunnel: w363 -> [w409 _]
          tunnel: w353 -> [w408 _]
          tunnel: [w405 w411] -> w364
          tunnel: w363 -> [_ w414]
          tunnel: w353 -> [_ w413]
          tunnel: w386 -> [w404 w412]
          tunnel: [w405 w411] -> w362
          tunnel: [w403 w410] -> w360
          frame False {
            n172 = Add(x=w404, y=3) -> (x+y=w406:i32)
            n173 = Replace Array Subset "Replace Array Subset"(array=w409, new element #1=w408, index #1=w404, new element #2=w408, index #2=w406) -> (w405:dbl[])
          }
          frame True {
            n174 = Replace Array Subset "Replace Array Subset"(array=w414, new element=w413, index=w412) -> (w411:dbl[])
          }
        }
        n175 = property class="Arr (strict)"(reference=w388, "Value"=w353) -> ()  [unwired: 1 in, 2 out]
        n176 = Array Subset "Array Subset"(array=w362, length=12) -> (w370:dbl[])  [unwired: 1 in]
        n177 = Multiply Array Elements(1:w370) -> (0:w371:dbl)
        n178 = Reshape Array "Reshape Array"(w370, 4 ("dimension size"), 3 ("dimension size")) -> (w367:dbl[][])
        n179 = for {
          tunnel: w367 -> [w415] mode=indexing
          tunnel: [w416] -> w366 mode=indexing
          n180 = Index Array(array=w415) -> ()  [unwired: 2 in, 2 out]
          n181 = Array To Cluster(array=w415) -> (cluster=w416:cluster{"[0]":dbl, "[1]":dbl})
        }
        n182 = Not Equal To 0?(x=w371) -> (x != 0?=w365:bool)
        "All fiducials recorded" <- w365
        n183 = property on="Manual Mode On" class="Bool (strict)"() -> ("Value"=w358:bool)  [unwired: 2 in, 2 out]
        n184 = case shown="True" w365 {
          tunnel: w364 -> [w420 w439]
          tunnel: w373 -> [_ _]
          tunnel: w366 -> [w422 w440]
          tunnel: w361 -> [_ w438]
          tunnel: w360 -> [w419 _]
          tunnel: w355 -> [w421 w437]
          tunnel: [w418 w436] -> w359
          tunnel: w358 -> [w417 w434]
          tunnel: w352 -> [_ w433]
          frame False {
            n185 = flat-sequence {
              tunnel: w422 -> [w426]
              tunnel: w421 -> [w425]
              tunnel: w420 -> [w424]
              tunnel: [w423] -> w418
              tunnel: w419 -> [w428]
              tunnel: w417 -> [w427]
              frame #0 {
                n186 = Bundle By Name(cluster=w425, "New Fiducials"=w424) -> (w423:T5)
                "XY Graph" <- w426
              }
              frame #1 {
                n187 = case shown="False" w428 {
                  selector: w428 -> [_ w432]
                  tunnel: w427 -> [w429 _]
                  frame False {
                    n188 = case shown="True" w429 {
                      selector: w429 -> [_ w431]
                      frame False {
                        n189 = property on="Go to CH8/FD2" class="Bool (strict)"("Val(Sgnl)"=TRUE ("Value (Signaling)")) -> ()  [unwired: 2 in, 2 out]
                      }
                      frame True {
                        n190 = property on="Enter Manual Mode" class="Bool (strict)"("Val(Sgnl)"=w431) -> ()  [unwired: 2 in, 2 out]
                      }
                    }
                  }
                  frame True {
                    n191 = property on="Predict fiducials" class="Bool (strict)"("Val(Sgnl)"=w432) -> ()  [unwired: 2 in, 2 out]
                  }
                }
              }
            }
          }
          frame True {
            n192 = flat-sequence {
              tunnel: w440 -> [w466]
              tunnel: w439 -> [w464]
              tunnel: w438 -> [w457]
              tunnel: w437 -> [w443]
              tunnel: [w442] -> w435
              tunnel: w433 -> [w441]
              tunnel: [w516] -> w436
              tunnel: w435 -> [w516]
              tunnel: w434 -> [w515]
              frame #0 {
                n193 = case shown="\"Module LD Bottom\"" w441 {
                  tunnel: ["calculate_center_adjY_axisX" ("function name") "calculate_center_adjY_axisX" ("function name") "calculate_center_adjY_axisX" ("function name") "calculate_center_adjX_axisY" ("function name") "calculate_center_adjX_axisY" ("function name") "calculate_center_adjX_axisY" ("function name") "calculate_center_adjY_axisY" ("function name") "calculate_center_adjX_axisY" ("function name") "calculate_center_adjX_axisY" ("function name") "calculate_center_adjX_axisY" ("function name") "calculate_center_adjY_axisY" ("function name") "calculate_center" ("function name") "calculate_center" ("function name") "calculate_center" ("function name") "calculate_center" ("function name") "calculate_center" ("function name")] -> w460
                  tunnel: [28.0 -2.0 0.0 -1.38 21.0 2.0 45.14 41.64 -41.64 49.78 -45.14 0.0 0.0 0.0 0.0 0.0] -> w459
                  tunnel: [1 0 1 1 1 1 1 1 1 1 0 1 1 1 1 1] -> w458
                  frame "Module LD Right" {
                  }
                  frame "Module LD Left " {
                  }
                  frame "Module LD Five" {
                  }
                  frame "Module LD Bottom" {
                  }
                  frame "Module HD Top" {
                  }
                  frame "Module LD Top" {
                  }
                  frame "Protomodule LD Right" {
                  }
                  frame "Protomodule LD Top" {
                  }
                  frame "Protomodule LD Bottom" {
                  }
                  frame "Protomodule HD Top" {
                  }
                  frame "Protomodule LD Left" {
                  }
                  frame "Protomodule LD Full", Default {
                  }
                  frame "Protomodule LD Five" {
                  }
                  frame "Protomodule HD Full" {
                  }
                  frame "Module LD Full" {
                  }
                  frame "Module HD Full" {
                  }
                }
                n194 = Index Array(array=w466) -> (element=w465:cluster{"[0]":dbl, "[1]":dbl})  [unwired: 1 in]
                n195 = Build Array (concatenate)(w466, w465) -> (w456:cluster{"[0]":dbl, "[1]":dbl}[])
                n196 = property on="XY Graph" class="XYGraph (strict)"("Val(Sgnl)"=w456) -> ()  [unwired: 2 in, 2 out]
                n197 = call "Base File Path.vi"() -> ("Paths Out"=w451:T10)  [unwired: 11 in]
                n198 = Unbundle By Name(w451) -> ("Components Folder"=w449:path)
                n199 = call "Get Python Version.vi"() -> ("Python Version"=w445:string, "error out"=w444:errorcluster)  [unwired: 10 in]
                n200 = Build Path(base path=w449, name or relative path=path "Calculate Component Center.py") -> (appended path=w448:path)
                n201 = Open Python Session(python version=w445, 3:w444) -> (session out=w455:refnum<k35>, error out=w453:errorcluster)  [unwired: 1 in]
                n202 = node(w455, w448, w460, w453, dbl[][] [], w464, w457, w459, w458) -> (w454:refnum<k35>, w452:errorcluster, w446:dbl[][])  [unwired: 4 in, 2 out]
                n203 = Close Python Session(session in=w454, error in=w452) -> ()  [unwired: 1 out]
                n204 = Index Array(array=w446) -> (element #1=w461:dbl[], element #2=w462:dbl[], element #3=w463:dbl[])  [unwired: 6 in]
                "XYZTheta" <- w461
                "CH1 XYZ" <- w462
                "Sensor ID Location" <- w463
                n205 = Bundle By Name(cluster=w443, "New Fiducials"=w464, "XYZTheta"=w461, "CH1 Location"=w462, "Sensor ID Location"=w463, "Position"=w457) -> (w442:T5)
              }
              frame #1 {
                n206 = case shown="False" w515 {
                  selector: w515 -> [_ w518]
                  frame False {
                    n207 = property on="Go to CH1" class="Bool (strict)"("Val(Sgnl)"=TRUE ("Value (Signaling)")) -> ()  [unwired: 2 in, 2 out]
                  }
                  frame True {
                    n208 = property on="Enter Manual Mode" class="Bool (strict)"("Val(Sgnl)"=w518) -> ()  [unwired: 2 in, 2 out]
                  }
                }
              }
            }
          }
        }
      }
      event "Predict fiducials": Value Change {
        n209 = event-data() -> ()  [unwired: 1 in, 6 out]
        n210 = Unbundle By Name(w522) -> ("Past Fiducials"=w523:dbl[][], "New Fiducials"=w526:dbl[], "Position"=w524:i32, "initial rotation"=w520:dbl[], "Assembly Type"=w519:string)
        n211 = flat-sequence {
          tunnel: w526 -> [w538]
          tunnel: [w538] -> w525
          tunnel: w524 -> [w539]
          tunnel: w523 -> [w537]
          tunnel: w522 -> [w532]
          tunnel: [w531] -> w521
          tunnel: w520 -> [w530]
          tunnel: w519 -> [w529]
          tunnel: w525 -> [w550]
          frame #0 {
            n212 = call "Base File Path.vi"() -> ("Paths Out"=w548:T10)  [unwired: 11 in]
            n213 = Unbundle By Name(w548) -> ("Components Folder"=w544:path)
            n214 = call "Get Python Version.vi"() -> ("Python Version"=w547:string, "error out"=w546:errorcluster)  [unwired: 10 in]
            n215 = Build Path(base path=w544, name or relative path=path "fiducial_prediction.py") -> (appended path=w542:path)
            n216 = Open Python Session(python version=w547, 3:w546) -> (session out=w543:refnum<k35>, error out=w540:errorcluster)  [unwired: 1 in]
            n217 = node(w543, w542, "fiducial_prediction" ("function name"), w540, dbl[][] [], w529, w539, w538, w537, w530) -> (w534:refnum<k35>, w533:errorcluster, w536:dbl[][])  [unwired: 5 in, 2 out]
            "predicted fiducials" <- w536
            n218 = Close Python Session(session in=w534, error in=w533) -> ()  [unwired: 1 out]
            n219 = Bundle By Name(cluster=w532, "Past Fiducials"=w536) -> (w531:T5)
          }
          frame #1 {
            n220 = property on="Manual Mode On" class="Bool (strict)"() -> ("Value"=w549:bool)  [unwired: 2 in, 2 out]
            n221 = case shown="False" w549 {
              selector: w549 -> [_ w561]
              tunnel: w550 -> [w556 _]
              frame False {
                n222 = Search 1D Array(1D array=w556, element=0.0) -> (index of element=w554:i32)  [unwired: 1 in]
                n223 = Divide(x=w554, y=3) -> (x/y=w552:dbl)
                n224 = case shown="0, Default" w552 {
                  tunnel: TRUE ("Value (Signaling)") -> [w557 w558 w559 w560]
                  frame 0, Default {
                    n225 = property on="Go to CH1/FD1" class="Bool (strict)"("Val(Sgnl)"=w557) -> ()  [unwired: 2 in, 2 out]
                  }
                  frame 1 {
                    n226 = property on="Go to CH191/FD5" class="Bool (strict)"("Val(Sgnl)"=w558) -> ()  [unwired: 2 in, 2 out]
                  }
                  frame 2 {
                    n227 = property on="Go to CH8/FD2" class="Bool (strict)"("Val(Sgnl)"=w559) -> ()  [unwired: 2 in, 2 out]
                  }
                  frame 3 {
                    n228 = property on="Go to CH197/FD4" class="Bool (strict)"("Val(Sgnl)"=w560) -> ()  [unwired: 2 in, 2 out]
                  }
                }
              }
              frame True {
                n229 = property on="Enter Manual Mode" class="Bool (strict)"("Val(Sgnl)"=w561) -> ()  [unwired: 2 in, 2 out]
              }
            }
          }
        }
        n230 = property on="Predict fiducials" class="Bool (strict)"("Value"=FALSE ("Predict fiducials")) -> ()  [unwired: 2 in, 2 out]
      }
      event "Focus": Value Change {
        n231 = event-data() -> ()  [unwired: 1 in, 6 out]
        n232 = Divide(x="number of focus steps", y=2) -> (x/y=w576:dbl)
        n233 = Multiply(x=w576, y="Focus step size") -> (x*y=w574:dbl)
        n234 = call "Joystick.vi"("Joystick"=FALSE, "Gantry In"=w573) -> ("Gantry Out"=w567:refnum<k24>)  [unwired: 8 in, 1 out]
        n235 = Negate(x=w574) -> (-x=w568:dbl)
        n236 = call "Z Go.vi"("Increment"=TRUE, "Return Immediately"=FALSE ("Increment"), "Speed In"=1.0 ("Speed"), "Position In"=w568, "Gantry In"=w567) -> ("error out"=w565:errorcluster, "Gantry Out"=w566:refnum<k24>)  [unwired: 3 in, 2 out]
        n237 = for {
          N: "number of focus steps" -> [_]
          tunnel: [w593] -> w587 mode=indexing
          tunnel: w565 -> [w592]
          tunnel: [w590] -> w580
          shift-right: [w594] -> w581
          shift-left: w566 -> [w596]
          tunnel: "Focus step size" -> [w589]
          n238 = flat-sequence {
            tunnel: w596 -> [w604]
            tunnel: [w603] -> w595
            tunnel: w592 -> [w602]
            tunnel: [w601] -> w591
            tunnel: w589 -> [w599]
            tunnel: w595 -> [w613]
            tunnel: [w612] -> w594
            tunnel: [w611] -> w593
            tunnel: w591 -> [w607]
            tunnel: [w606] -> w590
            frame #0 {
              n239 = call "Z Go.vi"("Increment"=TRUE, "Return Immediately"=FALSE ("Increment"), "error in (no error)"=w602, "Speed In"=0.1 ("Speed"), "Position In"=w599, "Gantry In"=w604) -> ("error out"=w601:errorcluster, "Gantry Out"=w603:refnum<k24>)  [unwired: 2 in, 2 out]
            }
            frame #1 {
              n240 = call "Get Current Position.vi"("error in (no error)"=w607, "Gantry In"=w613) -> ("error out"=w606:errorcluster, "XYZTheta Out"=w610:dbl[], "Gantry Out"=w612:refnum<k24>)  [unwired: 7 in]
              n241 = local read "Average Strength"() -> (w605:dbl)
              n242 = Delete From Array(array=w610, index=2) -> (deleted portion=w608:dbl)  [unwired: 1 in, 1 out]
              n243 = Build Array(w605, w608) -> (w611:dbl[])
            }
          }
        }
        n244 = Transpose 2D Array(2D array=w587) -> (transposed array=w586:dbl[][])
        n245 = Index Array(array=w586) -> (element #2=w585:dbl[])  [unwired: 4 in, 1 out]
        n246 = Index Array(array=w586) -> (element=w588:dbl[])  [unwired: 2 in]
        n247 = Array Max & Min(array=w588) -> (max index (indices)=w584:i32)  [unwired: 3 out]
        n248 = Index Array(array=w585, index=w584) -> (element=w583:dbl)
        n249 = call "Z Go.vi"("Increment"=FALSE, "Return Immediately"=FALSE ("Increment"), "error in (no error)"=w580, "Speed In"=15.0 ("Speed"), "Position In"=w583, "Gantry In"=w581) -> ("Gantry Out"=w572:refnum<k24>)  [unwired: 2 in, 3 out]
      }
      event "Joystick": Value Change {
        n250 = event-data() -> ()  [unwired: 1 in, 6 out]
        n251 = call "Joystick.vi"("Joystick"="Joystick", "Gantry In"=w616) -> ("Gantry Out"=w614:refnum<k24>)  [unwired: 8 in, 1 out]
      }
      event "Go to Center": Value Change {
        n252 = event-data() -> ()  [unwired: 1 in, 6 out]
        n253 = Unbundle By Name(w625) -> ("XYZTheta"=w626:dbl[])
        n254 = control-ref of="Joystick"() -> (w622:refnum<vi>)
        n255 = property class="Bool (strict)"(reference=w622) -> (reference out=w623:refnum<vi>, "Value"=w624:bool)  [unwired: 1 in, 1 out]
        n256 = case shown="True" w624 {
          selector: w624 -> [_ w641]
          tunnel: w621 -> [w635 w638]
          tunnel: [w635 w637] -> w620
          tunnel: w623 -> [_ w640]
          frame False {
          }
          frame True {
            n257 = Not(x=w641) -> (.not. x?=w636:bool)
            n258 = call "Joystick.vi"("Joystick"=w636, "Gantry In"=w638) -> ("error out"=w639:errorcluster, "Gantry Out"=w637:refnum<k24>)  [unwired: 8 in]
            n259 = property class="Bool (strict)"(reference=w640, error in=w639, "Value"=w636) -> ()  [unwired: 2 out]
          }
        }
        n260 = flat-sequence {
          tunnel: w626 -> [w631]
          tunnel: w620 -> [w630]
          tunnel: [w629] -> w618
          tunnel: [w633] -> w619
          tunnel: w618 -> [w633]
          frame #0 {
            w627 = T7."Disabled and Grayed Out" ("Disabled")
            n261 = call "ClearXYZTheta Go.vi"("XYZTheta In"=w631, "Gantry In"=w630) -> ("Gantry Out"=w629:refnum<k24>)  [unwired: 7 in, 2 out]
            n262 = property on="Record CH191/FD5" class="Bool (strict)"("DisabledEnum"=w627) -> ()  [unwired: 2 in, 2 out]
            n263 = property on="Go to CH1/FD1" class="Bool (strict)"("DisabledEnum"=w627) -> ()  [unwired: 2 in, 2 out]
            n264 = property on="Go to CH191/FD5" class="Bool (strict)"("DisabledEnum"=w627) -> ()  [unwired: 2 in, 2 out]
            n265 = property on="Go to CH1" class="Bool (strict)"("DisabledEnum"=w627) -> ()  [unwired: 2 in, 2 out]
            n266 = property on="Record CH8/FD2" class="Bool (strict)"("DisabledEnum"=w627) -> ()  [unwired: 2 in, 2 out]
            n267 = property on="Stop Program" class="Bool"("DisabledEnum"=w627) -> ()  [unwired: 2 in, 2 out]
            n268 = property on="Go to CH197/FD4" class="Bool (strict)"("DisabledEnum"=w627) -> ()  [unwired: 2 in, 2 out]
            n269 = property on="Go to CH8/FD2" class="Bool (strict)"("DisabledEnum"=w627) -> ()  [unwired: 2 in, 2 out]
            n270 = property on="Go to Sensor ID" class="Bool (strict)"("DisabledEnum"=w627) -> ()  [unwired: 2 in, 2 out]
            n271 = property on="Record CH1/FD1" class="Bool (strict)"("DisabledEnum"=w627) -> ()  [unwired: 2 in, 2 out]
            n272 = property on="Go to Center" class="Bool"("DisabledEnum"=w627) -> ()  [unwired: 2 in, 2 out]
            n273 = property on="Record CH197/FD4" class="Bool (strict)"("DisabledEnum"=w627) -> ()  [unwired: 2 in, 2 out]
            n274 = property on="Instructions" class="Str"("Val(Sgnl)"="Moving to component center. Wait for movement to stop." ("Value (Signaling)")) -> ()  [unwired: 2 in, 2 out]
          }
          frame #1 {
            n275 = property on="Manual Mode On" class="Bool (strict)"() -> ("Value"=w632:bool)  [unwired: 2 in, 2 out]
            n276 = case shown="True" w632 {
              selector: w632 -> [_ w634]
              frame False {
              }
              frame True {
                n277 = property on="Enter Manual Mode" class="Bool (strict)"("Val(Sgnl)"=w634) -> ()  [unwired: 2 in, 2 out]
              }
            }
          }
        }
      }
      event "Go to CH1": Value Change {
        n278 = event-data() -> ()  [unwired: 1 in, 6 out]
        n279 = Unbundle By Name(w650) -> ("CH1 Location"=w651:dbl[])
        n280 = property on="Go to CH1" class="Bool (strict)"("Value"=FALSE ("Go to CH1")) -> ()  [unwired: 2 in, 2 out]
        n281 = control-ref of="Joystick"() -> (w647:refnum<vi>)
        n282 = property class="Bool (strict)"(reference=w647) -> (reference out=w648:refnum<vi>, "Value"=w649:bool)  [unwired: 1 in, 1 out]
        n283 = case shown="True" w649 {
          selector: w649 -> [_ w672]
          tunnel: w646 -> [w666 w669]
          tunnel: [w666 w668] -> w645
          tunnel: w648 -> [_ w671]
          frame False {
          }
          frame True {
            n284 = Not(x=w672) -> (.not. x?=w667:bool)
            n285 = call "Joystick.vi"("Joystick"=w667, "Gantry In"=w669) -> ("error out"=w670:errorcluster, "Gantry Out"=w668:refnum<k24>)  [unwired: 8 in]
            n286 = property class="Bool (strict)"(reference=w671, error in=w670, "Value"=w667) -> ()  [unwired: 2 out]
          }
        }
        n287 = flat-sequence {
          tunnel: w651 -> [w656]
          tunnel: w645 -> [w655]
          tunnel: [w654] -> w642
          tunnel: [w661] -> w644
          tunnel: w642 -> [w661]
          frame #0 {
            w652 = T7."Disabled and Grayed Out" ("Disabled")
            n288 = call "ClearXYZTheta Go.vi"("XYZTheta In"=w656, "Gantry In"=w655) -> ("Gantry Out"=w654:refnum<k24>)  [unwired: 7 in, 2 out]
            n289 = property on="Record CH191/FD5" class="Bool (strict)"("DisabledEnum"=w652) -> ()  [unwired: 2 in, 2 out]
            n290 = property on="Stop Program" class="Bool"("DisabledEnum"=w652) -> ()  [unwired: 2 in, 2 out]
            n291 = property on="Go to CH1/FD1" class="Bool (strict)"("DisabledEnum"=w652) -> ()  [unwired: 2 in, 2 out]
            n292 = property on="Go to CH1" class="Bool (strict)"("DisabledEnum"=w652) -> ()  [unwired: 2 in, 2 out]
            n293 = property on="Record CH1/FD1" class="Bool (strict)"("DisabledEnum"=w652) -> ()  [unwired: 2 in, 2 out]
            n294 = property on="Go to Center" class="Bool"("DisabledEnum"=w652) -> ()  [unwired: 2 in, 2 out]
            n295 = property on="Go to CH191/FD5" class="Bool (strict)"("DisabledEnum"=w652) -> ()  [unwired: 2 in, 2 out]
            n296 = property on="Go to Sensor ID" class="Bool (strict)"("DisabledEnum"=w652) -> ()  [unwired: 2 in, 2 out]
            n297 = property on="Go to CH197/FD4" class="Bool (strict)"("DisabledEnum"=w652) -> ()  [unwired: 2 in, 2 out]
            n298 = property on="Record CH197/FD4" class="Bool (strict)"("DisabledEnum"=w652) -> ()  [unwired: 2 in, 2 out]
            n299 = property on="Go to CH8/FD2" class="Bool (strict)"("DisabledEnum"=w652) -> ()  [unwired: 2 in, 2 out]
            n300 = property on="Record CH8/FD2" class="Bool (strict)"("DisabledEnum"=w652) -> ()  [unwired: 2 in, 2 out]
            n301 = property on="Instructions" class="Str"("Val(Sgnl)"="Moving to CH1. Wait for movement to stop." ("Value (Signaling)")) -> ()  [unwired: 2 in, 2 out]
          }
          frame #1 {
            n302 = Two Button Dialog(message="Is CH1 visible?", 1:"No" ("F button name (\"Cancel\")"), 2:"Yes" ("T button name (\"OK\")")) -> (T button?=w657:bool)
            "CH1 correct?" <- w657
            n303 = case shown="True" w657 {
              frame False {
                n304 = property on="Enter Manual Mode" class="Bool (strict)"("Val(Sgnl)"=TRUE ("Value (Signaling)")) -> ()  [unwired: 2 in, 2 out]
              }
              frame True {
                n305 = property on="Manual Mode On" class="Bool (strict)"() -> ("Value"=w663:bool)  [unwired: 2 in, 2 out]
                n306 = case shown="False" w663 {
                  selector: w663 -> [_ w665]
                  frame False {
                    n307 = property on="Go to Sensor ID" class="Bool (strict)"("Val(Sgnl)"=TRUE ("Go to Sensor ID")) -> ()  [unwired: 2 in, 2 out]
                  }
                  frame True {
                    n308 = property on="Enter Manual Mode" class="Bool (strict)"("Val(Sgnl)"=w665) -> ()  [unwired: 2 in, 2 out]
                  }
                }
              }
            }
          }
        }
      }
      event "Enter Manual Mode": Value Change {
        w679 = T7."Enabled" ("Disabled")
        n309 = event-data() -> ()  [unwired: 1 in, 6 out]
        n310 = case shown="True" w677 {
          tunnel: [T7."Disabled and Grayed Out" ("Disabled") T7."Enabled" ("Disabled")] -> w678
          frame False {
          }
          frame True {
          }
        }
        n311 = property on="Enter Manual Mode" class="Bool (strict)"("Value"=FALSE ("Enter Manual Mode")) -> ()  [unwired: 2 in, 2 out]
        n312 = property on="Go to CH1" class="Bool (strict)"("DisabledEnum"=w679) -> ()  [unwired: 2 in, 2 out]
        n313 = property on="Go to Sensor ID" class="Bool (strict)"("DisabledEnum"=w679) -> ()  [unwired: 2 in, 2 out]
        n314 = property on="Record CH1/FD1" class="Bool (strict)"("DisabledEnum"=w679) -> ()  [unwired: 2 in, 2 out]
        n315 = property on="Go to CH8/FD2" class="Bool (strict)"("DisabledEnum"=w679) -> ()  [unwired: 2 in, 2 out]
        n316 = property on="Go to Center" class="Bool"("DisabledEnum"=w679) -> ()  [unwired: 2 in, 2 out]
        n317 = property on="Record CH8/FD2" class="Bool (strict)"("DisabledEnum"=w679) -> ()  [unwired: 2 in, 2 out]
        n318 = property on="Go to CH1/FD1" class="Bool (strict)"("DisabledEnum"=w679) -> ()  [unwired: 2 in, 2 out]
        n319 = property on="Stop Program" class="Bool"("DisabledEnum"=w679) -> ()  [unwired: 2 in, 2 out]
        n320 = property on="Instructions" class="Str"("Val(Sgnl)"="Now in manual mode." ("Value (Signaling)")) -> ()  [unwired: 2 in, 2 out]
        n321 = case shown="True" "Enter Manual Mode" {
          selector: "Enter Manual Mode" -> [_ w681]
          frame False {
          }
          frame True {
            "Manual Mode On" <- w681
          }
        }
        n322 = property on="Go to CH191/FD5" class="Bool (strict)"("DisabledEnum"=w678) -> ()  [unwired: 2 in, 2 out]
        n323 = property on="Record CH191/FD5" class="Bool (strict)"("DisabledEnum"=w678) -> ()  [unwired: 2 in, 2 out]
        n324 = property on="Go to CH197/FD4" class="Bool (strict)"("DisabledEnum"=w678) -> ()  [unwired: 2 in, 2 out]
        n325 = property on="Record CH197/FD4" class="Bool (strict)"("DisabledEnum"=w678) -> ()  [unwired: 2 in, 2 out]
      }
      event "Go to Sensor ID": Value Change {
        n326 = event-data() -> ()  [unwired: 1 in, 6 out]
        n327 = flat-sequence {
          tunnel: w688 -> [w690]
          tunnel: w687 -> [w692]
          tunnel: [w691] -> w684
          tunnel: [w826] -> w686
          tunnel: w684 -> [w826]
          frame #0 {
            n328 = Unbundle By Name(w690) -> ("Protomodule?"=w689:bool)
            n329 = case shown="True" w689 {
              tunnel: w690 -> [_ w745]
              tunnel: w692 -> [w693 w744]
              tunnel: [w693 w743] -> w691
              frame False {
              }
              frame True {
                w694 = T7."Disabled and Grayed Out" ("Disabled")
                # "Will replace this with automatic checking"
                n330 = Unbundle By Name(w745) -> ("Sensor ID Location"=w742:dbl[], "XYZTheta"=w741:dbl[], "Position"=w740:i32)
                n331 = Index Array(array=w741, index=3) -> (element=w704:dbl)
                n332 = Equal To 0?(x=w740) -> (x = 0?=w706:bool)
                n333 = case shown="True" w706 {
                  tunnel: [0.44 ("r") -0.44 ("r")] -> w705
                  frame False {
                  }
                  frame True {
                  }
                }
                n334 = Array Subset(array=w742, length=2) -> (w724:dbl[])  [unwired: 1 in]
                n335 = Add(x=w704, y=1.5707963267948966) -> (x+y=w731:dbl)
                n336 = property on="Instructions" class="Str"("Val(Sgnl)"="Now determining sensor ID." ("Value (Signaling)")) -> ()  [unwired: 2 in, 2 out]
                n337 = property on="Go to CH1" class="Bool (strict)"("DisabledEnum"=w694) -> ()  [unwired: 2 in, 2 out]
                n338 = call "XY Go.vi"("return immediately"=FALSE, "Speed"=100.0, "XY In"=w724, "Gantry In"=w744) -> ("error out"=w709:errorcluster, "XY Out"=w723:dbl[], "Gantry Out"=w727:refnum<k24>)  [unwired: 5 in]
                n339 = property on="Go to CH1/FD1" class="Bool (strict)"("DisabledEnum"=w694) -> ()  [unwired: 2 in, 2 out]
                n340 = property on="Go to CH191/FD5" class="Bool (strict)"("DisabledEnum"=w694) -> ()  [unwired: 2 in, 2 out]
                n341 = property on="Record CH8/FD2" class="Bool (strict)"("DisabledEnum"=w694) -> ()  [unwired: 2 in, 2 out]
                n342 = property on="Go to CH197/FD4" class="Bool (strict)"("DisabledEnum"=w694) -> ()  [unwired: 2 in, 2 out]
                n343 = property on="Go to CH8/FD2" class="Bool (strict)"("DisabledEnum"=w694) -> ()  [unwired: 2 in, 2 out]
                n344 = property on="Record CH1/FD1" class="Bool (strict)"("DisabledEnum"=w694) -> ()  [unwired: 2 in, 2 out]
                n345 = property on="Record CH191/FD5" class="Bool (strict)"("DisabledEnum"=w694) -> ()  [unwired: 2 in, 2 out]
                n346 = property on="Go to Center" class="Bool"("DisabledEnum"=w694) -> ()  [unwired: 2 in, 2 out]
                n347 = property on="Go to Sensor ID" class="Bool (strict)"("DisabledEnum"=w694) -> ()  [unwired: 2 in, 2 out]
                n348 = property on="Record CH197/FD4" class="Bool (strict)"("DisabledEnum"=w694) -> ()  [unwired: 2 in, 2 out]
                n349 = property on="Stop Program" class="Bool"("DisabledEnum"=w694) -> ()  [unwired: 2 in, 2 out]
                n350 = for {
                  N: 5 -> [_]
                  shift-right: [w749] -> _
                  shift-left: w723 -> [w753]
                  shift-right: [w752] -> _
                  shift-left: w731 -> [w752]
                  tunnel: [w749] -> w730 mode=indexing
                  shift-right: [w748] -> _
                  shift-left: w705 -> [w748]
                  n351 = in-place {
                    in-place-border: w752 -> [w755]
                    in-place-border: [w755] -> _
                    in-place-border: w748 -> [w754]
                    n352 = in-place-array #2(w753, 0, 1) -> (w761:dbl, w760:dbl)
                    n353 = Polar To Re/Im(2:w755, 3:w754) -> (0:w758:dbl, 1:w759:dbl)
                    n354 = Add(x=w761, y=w759) -> (x+y=w757:dbl)
                    n355 = Add(x=w760, y=w758) -> (x+y=w756:dbl)
                    n356 = in-place-array #2(w757, w756) -> (w749:dbl[])  [unwired: 2 out]
                  }
                }
                n357 = call "Base File Path.vi"() -> ("Paths Out"=w737:T10)  [unwired: 11 in]
                n358 = Unbundle By Name(w737) -> ("Components Folder"=w735:path)
                n359 = Build Path(base path=w735, name or relative path=path "temp") -> (appended path=w734:path)
                n360 = Build Array (concatenate)(w723, w730) -> (w728:dbl[][])
                n361 = Create Folder(path (use dialog)=w734, error in=w709) -> (created path=w733:path, error out=w708:errorcluster)  [unwired: 1 in, 1 out]
                n362 = for {
                  shift-right: [w776] -> w743
                  shift-left: w727 -> [w777]
                  shift-right: [w772] -> w710
                  shift-left: w733 -> [w772]
                  tunnel: w728 -> [w770] mode=indexing
                  shift-right: [w766] -> w707
                  shift-left: w708 -> [w769]
                  tunnel: [w762] -> w702 mode=indexing
                  i -> [w773]
                  n363 = flat-sequence {
                    tunnel: w777 -> [w784]
                    tunnel: [w781] -> w775
                    tunnel: w770 -> [w780]
                    tunnel: w769 -> [w779]
                    tunnel: [w778] -> w767
                    tunnel: w775 -> [w795]
                    tunnel: [w795] -> w774
                    tunnel: w773 -> [w791]
                    tunnel: w772 -> [w788]
                    tunnel: [w787] -> w771
                    tunnel: [w785] -> w768
                    tunnel: w767 -> [w785]
                    tunnel: w774 -> [w801]
                    tunnel: w771 -> [w796]
                    tunnel: w768 -> [w799]
                    tunnel: [w801] -> w765
                    tunnel: [w798] -> w764
                    tunnel: [w796] -> w763
                    tunnel: [w803] -> w766
                    tunnel: [w806] -> w776
                    tunnel: w765 -> [w806]
                    tunnel: w764 -> [w804]
                    tunnel: w763 -> [w805]
                    tunnel: [w802] -> w762
                    frame #0 {
                      n364 = call "XY Go.vi"("return immediately"=FALSE, "error in (no error)"=w779, "Speed"=100.0, "XY In"=w780, "Gantry In"=w784) -> ("error out"=w778:errorcluster, "Gantry Out"=w781:refnum<k24>)  [unwired: 4 in, 1 out]
                    }
                    frame #1 {
                      n365 = Wait (ms)(milliseconds to wait=u32 1000) -> ()  [unwired: 1 out]
                      n366 = Number To Decimal String(number=w791) -> (decimal integer string=w793:string)  [unwired: 1 in]
                      n367 = Concatenate Strings("temp" ("string"), w793, ".bmp" ("string")) -> (w794:string)
                      n368 = String To Path(string=w794) -> (path=w792:path)
                      n369 = Build Path(base path=w788, name or relative path=w792) -> (appended path=w787:path)
                    }
                    frame #2 {
                      n370 = local read "Image"() -> (w800:T6)
                      n371 = Wait (ms)(milliseconds to wait=u32 1000) -> ()  [unwired: 1 out]
                      n372 = call-poly "IMAQ Write File 2"("error in (no error)"=w799, "File Path"=w796, "Image"=w800) -> ("error out"=w798:errorcluster)  [unwired: 7 in, 1 out]
                    }
                    frame #3 {
                      n373 = disable-structure shown="Enabled" {
                        disable-tunnel: w805 -> [w813 w820]
                        disable-tunnel: w804 -> [w812 w819]
                        disable-tunnel: [w811 w818] -> w803
                        disable-tunnel: [w809 w821] -> w802
                        frame Disabled {
                          n374 = call <vilib>:"Read BMP File.vi"("error in (no error)"=w812, "path to BMP file"=w813) -> ("error out"=w811:errorcluster, "image data"=w808:T9)  [unwired: 7 in, 1 out]
                          n375 = in-place {
                            n376 = in-place-cluster #3(w808) -> ("Rectangle"=w816:T8)
                            n377 = Divide(x=w816, y=T8 {"left"=2, "top"=2, "right"=2, "bottom"=2}) -> (x/y=w814:T11)
                            n378 = in-place-cluster #3("Rectangle"=w814) -> (w807:T9)
                          }
                          n379 = call <vilib>:"Draw Flattened Pixmap.vi"("image data"=w807, "picture"=picture data[5B]) -> ("new picture"=w809:picture)  [unwired: 7 in]
                        }
                        frame Enabled {
                          n380 = call "Resize Image to a Container 2012 NIVerified.vi"("error in (no error)"=w819, "image data"=T9 {"image type"=0, "image depth"=0, "image"=[], "mask"=[], "colors"=[], "Rectangle"={"left"=0, "top"=200, "right"=200, "bottom"=0}}, "Path to Image (PNG, JPEG, BMP)"=w820) -> ("error out"=w818:errorcluster, "Resized Image"=w821:picture)  [unwired: 6 in]
                        }
                      }
                    }
                  }
                }
                "Sensor ID" <- w702
                n381 = call "Base File Path.vi"() -> ("Paths Out"=w718:T10)  [unwired: 11 in]
                n382 = Unbundle By Name(w718) -> ("Components Folder"=w717:path)
                n383 = call "Get Python Version.vi"("error in (no error)"=w707) -> ("Python Version"=w714:string, "error out"=w713:errorcluster)  [unwired: 9 in]
                n384 = Build Path(base path=w717, name or relative path=path "SensorID.py") -> (appended path=w716:path)
                n385 = Open Python Session(python version=w714, 3:w713) -> (session out=w722:refnum<k35>, error out=w720:errorcluster)  [unwired: 1 in]
                n386 = Path To String(path=w710) -> (string=w711:string)
                n387 = node(w722, w716, "read_sensor_ID" ("function name"), w720, "read_sensor_ID" ("string"), w711, w740, w704) -> (w721:refnum<k35>, w719:errorcluster, w701:string)  [unwired: 3 in, 2 out]
                "Sensor ID" <- w701
                n388 = Close Python Session(session in=w721, error in=w719) -> ()  [unwired: 1 out]
                n389 = Concatenate Strings(w701, " is the sensor ID. Does this match the input?" ("string")) -> (w699:string)
                n390 = Two Button Dialog(message=w699, 1:"No" ("F button name (\"Cancel\")"), 2:"Yes" ("T button name (\"OK\")")) -> (T button?=w696:bool)
                n391 = case shown="True" w696 {
                  frame False {
                  }
                  frame True {
                  }
                }
              }
            }
          }
          frame #1 {
            n392 = Two Button Dialog(message="Ready to Submit?", 1:"No" ("F button name (\"Cancel\")"), 2:"Yes" ("T button name (\"OK\")")) -> (T button?=w822:bool)
            n393 = case shown="True" w822 {
              selector: w822 -> [_ w828]
              frame False {
                n394 = property on="Enter Manual Mode" class="Bool (strict)"("Val(Sgnl)"=TRUE ("Value (Signaling)")) -> ()  [unwired: 2 in, 2 out]
              }
              frame True {
                n395 = property on="Auto Submit" class="Bool (strict)"("Val(Sgnl)"=w828) -> ()  [unwired: 2 in, 2 out]
              }
            }
          }
        }
        n396 = property on="Go to Sensor ID" class="Bool (strict)"("Value"=FALSE ("Go to Sensor ID")) -> ()  [unwired: 2 in, 2 out]
      }
    }
  }
  "Gantry Out" <- w28
  n397 = while {
    shift-right: [w847] -> _
    shift-left: w18 -> [w850]
    i -> [w843]
    stop <- w841 stop-if-true
    n398 = Or(x="Stop Program", y="Auto Submit") -> (x .or. y?=w837:bool)
    n399 = case shown="True" w837 {
      selector: w837 -> [w851 _]
      tunnel: [w851 w853] -> w841
      frame False {
      }
      frame True {
        n400 = property on="All fiducials recorded" class="Bool (strict)"() -> ("Value"=w855:bool)  [unwired: 2 in, 2 out]
        n401 = property on="CH1 correct?" class="Bool (strict)"() -> ("Value"=w854:bool)  [unwired: 2 in, 2 out]
        n402 = And(x=w855, y=w854) -> (x .and. y?=w852:bool)
        n403 = case shown="False" w852 {
          selector: w852 -> [w856 w858]
          tunnel: [w856 w858] -> w853
          frame False {
            n404 = One Button Dialog(message="At least one fiducial not recorded or component orientation not verified via CH1.") -> ()  [unwired: 1 in, 1 out]
          }
          frame True {
          }
        }
      }
    }
    "Program Stopped" <- w841
    n405 = Equal To 0?(x=w843) -> (x = 0?=w842:bool)
    n406 = call "Camera.vi"("Camera in"=w850, "Stop"=w841, "BCG Image Processing"="Image processing", "Machine Vision"="Machine Vision", "Camera settings"="Camera settings", "Loop 0"=w842, "Override presets"="Override presets") -> ("Camera out"=w847:refnum<class "Edmund Optics.lvclass">, "output cluster"=w836:T12, "pattern matching"=→"pattern matching":T1, "Image"=→"Image":T6, "Camera"=→"Camera":dbl[])  [unwired: 7 in, 1 out]
    n407 = Unbundle By Name(w836) -> ("Average Strength"=→"Average Strength":dbl, "Radius (Real-World)"=→"Radius (Real-World)":dbl, "Match found?"=→"Match found?":bool, "Global Report"=w832:T13)
    n408 = Unbundle By Name(w832) -> ("Standard Variation"=→"Standard Variation":sgl, "Maximal Value"=→"Maximal Value":sgl)
  }
